vi "Pressure.vi"(0 "VISA resource name":refnum<visa-resource-name>, 1 "baud rate (9600)":u32=9600, 2 "data bits (8)":u16=8 min=5 max=8 step=1, 3 "parity (0:none)":dbl, 4 "stop bits (10: 1 bit)":u16=10, 5 "flow control (0:none)":dbl, 6 "Recieve Data":bool, 7 "termination char\n(0xA = '\\n' = LF)":u8=13 format="%.0x") -> (13 "VISA resource name out":refnum<visa-resource-name>, 14 "output cluster":cluster{dbl, dbl, dbl}, 15 "output array":string[](array[string]), 16 "Response G1":string, 17 "Response G2":string, 18 "Response G3":string, 19 "error out":errorcluster)   [LabVIEW 2019]
uses:
  <vilib>/Instr/_visa.llb/VISA Configure Serial Port (Instr).vi
panel:
  out "bytes read 3":u32
  out "bytes read 2":u32
  out "bytes read":u32
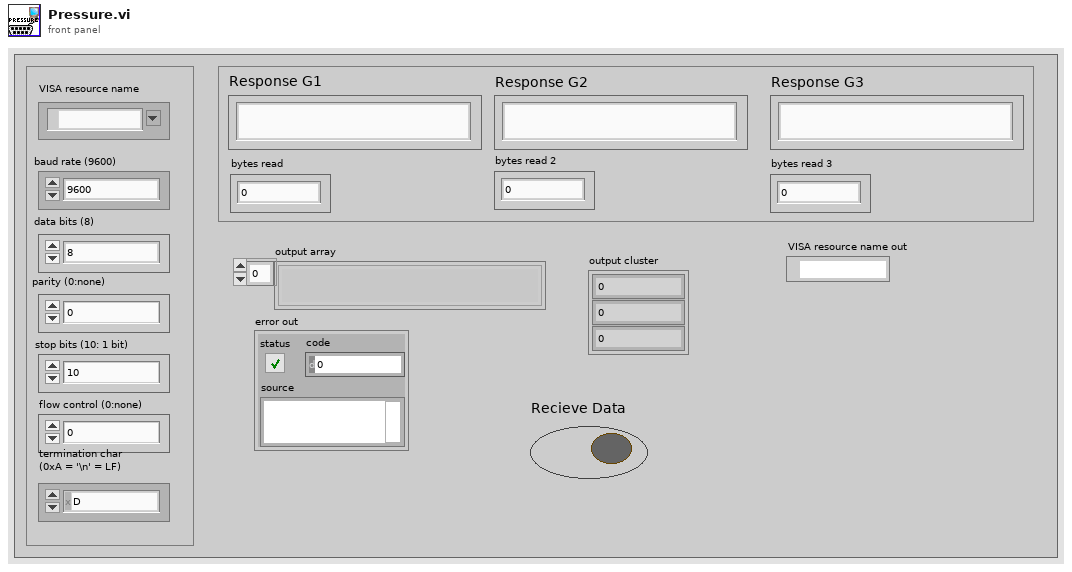
[diagram p1: front panel]
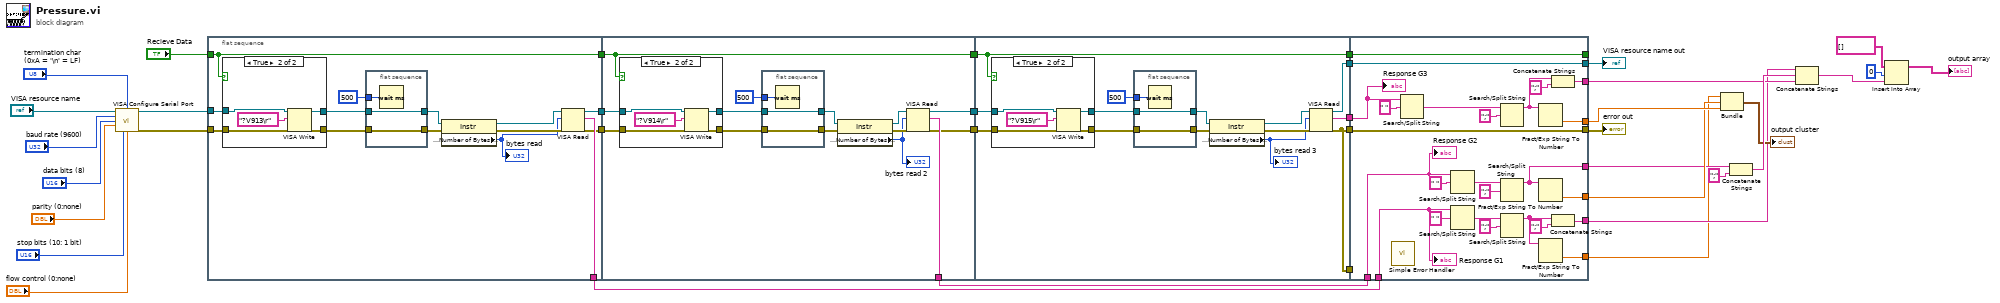
[diagram p0: block diagram]
diagram:
  n1 = call-poly "VISA Configure Serial Port"("VISA resource name"="VISA resource name", "termination char\n(0xA = '\\n' = LF)"="termination char\n(0xA = '\\n' = LF)", "baud rate (9600)"="baud rate (9600)", "data bits (8)"="data bits (8)", "parity (0:none)"="parity (0:none)", "stop bits (10: 1 bit)"="stop bits (10: 1 bit)", "flow control (0:none)"="flow control (0:none)") -> ("VISA resource name out"=w19:refnum<visa-resource-name>, "error out"=w18:errorcluster)  [unwired: 3 in, 4 out]
  n2 = flat-sequence {
    tunnel: [w42] -> w7
    tunnel: [w41] -> w31
    tunnel: [w40] -> w30
    tunnel: [w39] -> w29
    tunnel: "Recieve Data" -> [w39]
    tunnel: w18 -> [w47]
    tunnel: w19 -> [w46]
    tunnel: w31 -> [w71]
    tunnel: w30 -> [w70]
    tunnel: [w66] -> w8
    tunnel: [w64] -> w28
    tunnel: [w65] -> w27
    tunnel: w29 -> [w63]
    tunnel: [w63] -> w26
    tunnel: w28 -> [w97]
    tunnel: w27 -> [w96]
    tunnel: w26 -> [w87]
    tunnel: [w88] -> w15
    tunnel: [w90] -> w14
    tunnel: [w89] -> w13
    tunnel: [w88] -> w12
    tunnel: [w87] -> w11
    tunnel: [w133] -> _
    tunnel: [w134] -> w1
    tunnel: w15 -> [_]
    tunnel: w14 -> [w111]
    tunnel: w13 -> [w135]
    tunnel: w12 -> [w134]
    tunnel: w11 -> [w133]
    tunnel: [w127] -> w10
    tunnel: [w126] -> w9
    tunnel: w8 -> [w119]
    tunnel: w7 -> [w116]
    tunnel: [w115] -> w6
    tunnel: [w114] -> w5
    tunnel: [w113] -> w4
    tunnel: [w112] -> w3
    tunnel: [w111] -> w2
    frame #0 {
      n3 = case shown="True" w39 {
        tunnel: w47 -> [w53 w59]
        tunnel: w46 -> [w54 w58]
        tunnel: [w53 w57] -> w45
        tunnel: [w54 w55] -> w44
        frame False {
        }
        frame True {
          n4 = VISA Write(VISA resource name=w58, write buffer="?V913\r" ("Command"), error in (no error)=w59) -> (VISA resource name out=w55:refnum<visa-resource-name>, error out=w57:errorcluster)  [unwired: 1 out]
        }
      }
      n5 = flat-sequence {
        tunnel: w45 -> [w61]
        tunnel: [w61] -> w52
        tunnel: u32 500 ("delay before read (ms)") -> [w62]
        tunnel: w44 -> [w60]
        tunnel: [w60] -> w43
        frame #0 {
          n6 = Wait (ms)(milliseconds to wait=w62) -> ()  [unwired: 1 out]
        }
      }
      n7 = property class="Instr"(reference=w43, error in=w52) -> (reference out=w50:refnum<visa-resource-name>, error out=w49:errorcluster, "Serial Settings:Number of Bytes at Serial Port"=w48:u32)
      "bytes read" <- w48
      n8 = VISA Read(VISA resource name=w50, byte count=w48, error in (no error)=w49) -> (VISA resource name out=w41:refnum<visa-resource-name>, read buffer=w42:string, error out=w40:errorcluster)  [unwired: 1 out]
    }
    frame #1 {
      n9 = case shown="True" w63 {
        tunnel: w71 -> [w78 w82]
        tunnel: w70 -> [w77 w81]
        tunnel: [w78 w80] -> w69
        tunnel: [w77 w79] -> w68
        frame False {
        }
        frame True {
          n10 = VISA Write(VISA resource name=w82, write buffer="?V914\r" ("Command"), error in (no error)=w81) -> (VISA resource name out=w80:refnum<visa-resource-name>, error out=w79:errorcluster)  [unwired: 1 out]
        }
      }
      n11 = flat-sequence {
        tunnel: w68 -> [w85]
        tunnel: [w85] -> w67
        tunnel: u32 500 ("delay before read (ms)") -> [w86]
        tunnel: w69 -> [w84]
        tunnel: [w84] -> w73
        frame #0 {
          n12 = Wait (ms)(milliseconds to wait=w86) -> ()  [unwired: 1 out]
        }
      }
      n13 = property class="Instr"(reference=w73, error in=w67) -> (reference out=w76:refnum<visa-resource-name>, error out=w75:errorcluster, "Serial Settings:Number of Bytes at Serial Port"=w74:u32)
      "bytes read 2" <- w74
      n14 = VISA Read(VISA resource name=w76, byte count=w74, error in (no error)=w75) -> (VISA resource name out=w65:refnum<visa-resource-name>, read buffer=w66:string, error out=w64:errorcluster)  [unwired: 1 out]
    }
    frame #2 {
      n15 = case shown="True" w87 {
        tunnel: w97 -> [w101 w106]
        tunnel: w96 -> [w102 w105]
        tunnel: [w101 w104] -> w94
        tunnel: [w102 w103] -> w93
        frame False {
        }
        frame True {
          n16 = VISA Write(VISA resource name=w105, write buffer="?V915\r" ("Command"), error in (no error)=w106) -> (VISA resource name out=w103:refnum<visa-resource-name>, error out=w104:errorcluster)  [unwired: 1 out]
        }
      }
      n17 = flat-sequence {
        tunnel: u32 500 ("delay before read (ms)") -> [w110]
        tunnel: w94 -> [w109]
        tunnel: w93 -> [w108]
        tunnel: [w109] -> w92
        tunnel: [w108] -> w91
        frame #0 {
          n18 = Wait (ms)(milliseconds to wait=w110) -> ()  [unwired: 1 out]
        }
      }
      n19 = property class="Instr"(reference=w91, error in=w92) -> (reference out=w100:refnum<visa-resource-name>, error out=w99:errorcluster, "Serial Settings:Number of Bytes at Serial Port"=w98:u32)
      "bytes read 3" <- w98
      n20 = VISA Read(VISA resource name=w100, byte count=w98, error in (no error)=w99) -> (VISA resource name out=w90:refnum<visa-resource-name>, read buffer=w89:string, error out=w88:errorcluster)  [unwired: 1 out]
    }
    frame #3 {
      n21 = call <vilib>:"Simple Error Handler.vi"() -> ()  [unwired: 2 in, 8 out]
      n22 = Search/Split String(string=w135, search string/char (-)=" ") -> (match + rest of string=w132:string)  [unwired: 1 in, 2 out]
      n23 = Search/Split String(string=w119, search string/char (-)=" ") -> (match + rest of string=w124:string)  [unwired: 1 in, 2 out]
      n24 = Search/Split String(string=w116, search string/char (-)=" ") -> (match + rest of string=w125:string)  [unwired: 1 in, 2 out]
      n25 = Search/Split String(string=w132, search string/char (-)=";") -> (substring before match=w131:string)  [unwired: 1 in, 2 out]
      n26 = Search/Split String(string=w124, search string/char (-)=";") -> (substring before match=w113:string)  [unwired: 1 in, 2 out]
      n27 = Search/Split String(string=w125, search string/char (-)=";") -> (substring before match=w123:string)  [unwired: 1 in, 2 out]
      n28 = Fract/Exp String To Number(string=w131) -> (number=w126:dbl)  [unwired: 3 in, 1 out]
      n29 = Fract/Exp String To Number(string=w113) -> (number=w114:dbl)  [unwired: 3 in, 1 out]
      n30 = Fract/Exp String To Number(string=w123) -> (number=w112:dbl)  [unwired: 3 in, 1 out]
      n31 = Concatenate Strings(w131, ";" ("string")) -> (w127:string)
      n32 = Concatenate Strings(w123, ";" ("string")) -> (w115:string)
      "Response G3" <- w135
      "Response G1" <- w116
      "Response G2" <- w119
    }
  }
  n33 = Bundle(w3, w5, w9) -> (→"output cluster":cluster{dbl, dbl, dbl})  [unwired: 1 in]
  n34 = Concatenate Strings(w4, ";" ("string")) -> (w24:string)
  n35 = Concatenate Strings(w6, w24, w10) -> (w25:string)
  n36 = Insert Into Array(array=string[] [], index=0, new element=w25) -> (→"output array":string[])
  "error out" <- w1
  "VISA resource name out" <- w2
